vi "Menu Configurator.vi"() -> ()   [LabVIEW 2019, in "Menu Launcher Module.lvlib"]
uses:
  Menu Launcher Module/Menu Launcher Module.lvlib
  <vilib>/National Instruments/Tree Map/Tree Map Data.ctl
  <vilib>/picture/picture.llb/imagedata.ctl
  <vilib>/Utility/miscctls.llb/LVPointTypeDef.ctl
  <vilib>/Utility/miscctls.llb/LVMapReplaceAction.ctl
  <vilib>/National Instruments/Tree Map/API/List Roots.vi
  <vilib>/National Instruments/Tree Map/Utility/Into Tree Control Items.vi
  <vilib>/National Instruments/Tree Map/Tree Map.lvlib
panel:
  in  "New":bool
  in  "Edit":bool
  in  "Save":bool
  in  "Load":bool
  in  "Delete":bool
  in  "Add":bool
  in  "Menu Configuration":string(tree)
  in  "OK":bool
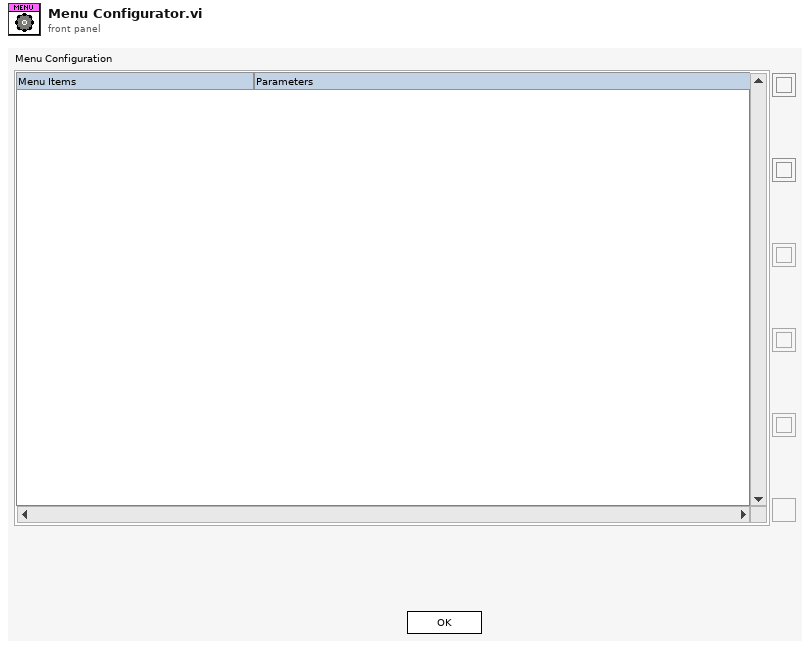
[diagram p1: front panel]
types:
  T1 = enum32{"Invalid", "Standard", "Closed", "Hidden", "Minimized", "Maximized"}
  T2 = enum32{"invalid app kind", "Development System", "Run Time System", "Student Edition", "Embedded LabVIEW", "Evaluation", "Custom"}
  T3 = typedef "Tree Map.lvlib/Tree Map Data.ctl" = map{string, cluster{"Child Paths Set":set{string}, "Name":string, "Data":string, "Attributes":map{string, string}}}
  T4 = typedef "LVPointTypeDef.ctl" = cluster{"Horizontal":i16, "Vertical":i16}
  T5 = enum16{"open", "replace", "create", "open or create", "replace or create", "replace or create with confirmation"}
  T6 = enum8{"Enabled", "Disabled", "Disabled and Grayed Out"}
  T7 = typedef "LVMapReplaceAction.ctl" = enum32{"Modify Entry only if found", "Add or Modify Entry", "Delete Entry"}
  T8 = cluster{"Core":cluster{"Current VI Reference":refnum<vi>, "Close Panel on Exit?":bool}, "SyncSols Menu":T3, "Data Node?":bool, "Path":string, "Selected Tag":string, "Data":string, "Current Path":path}
  T9 = cluster{"Current VI Reference":refnum<vi>, "Close Panel on Exit?":bool}
  T10 = typedef "imagedata.ctl" = cluster{"image type":i32, "image depth":i32, "image":u8[], "mask":u8[], "colors":u32[], "Rectangle":cluster{"left":i16, "top":i16, "right":i16, "bottom":i16}}
  T11 = cluster{"Left Cell String":string, "Child Text":string[], "Child Tag":string, "Item Indent":i32, "Child Only?":bool, "Glyph Index":i32}[]
  T12 = cluster{"Child Paths Set":set{string}, "Name":string, "Data":string, "Attributes":map{string, string}}
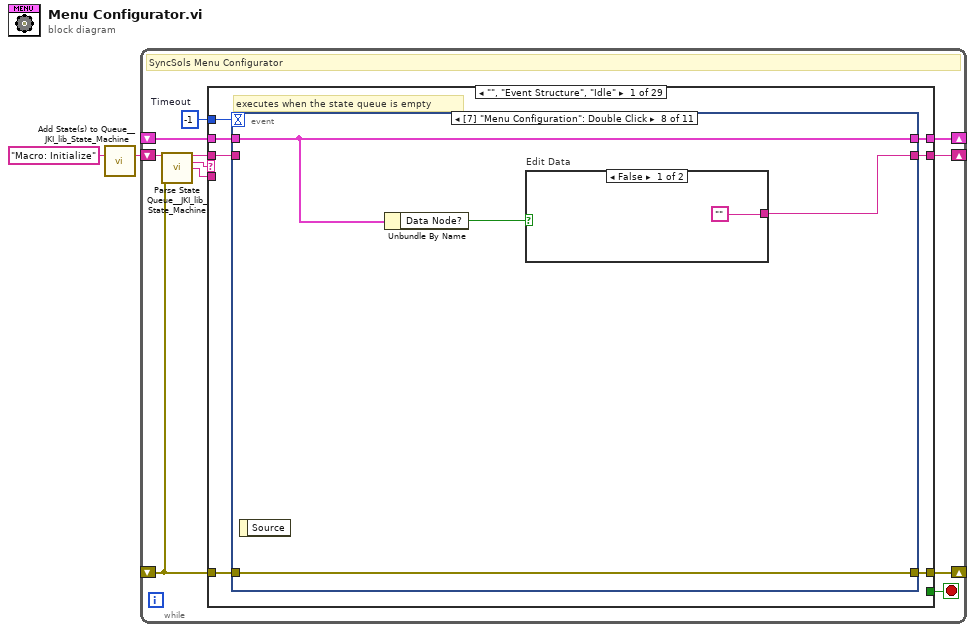
[diagram p0: block diagram]
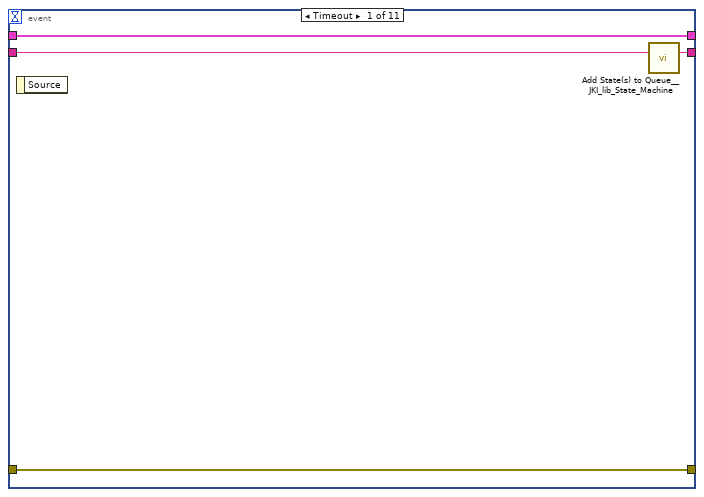
[diagram p2: hidden frame]
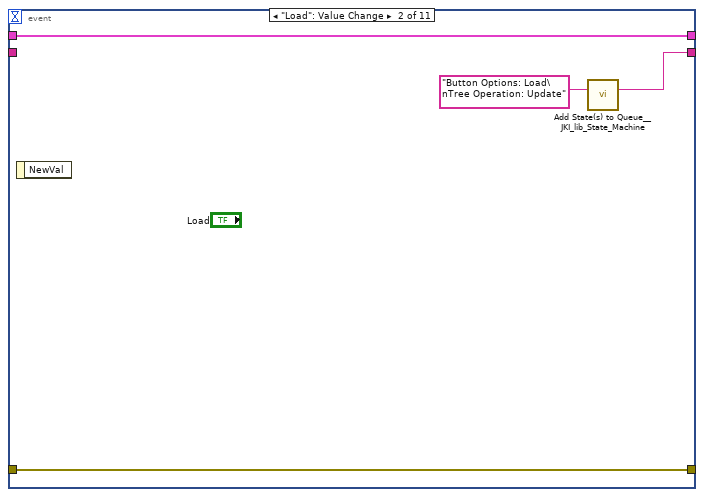
[diagram p3: hidden frame]
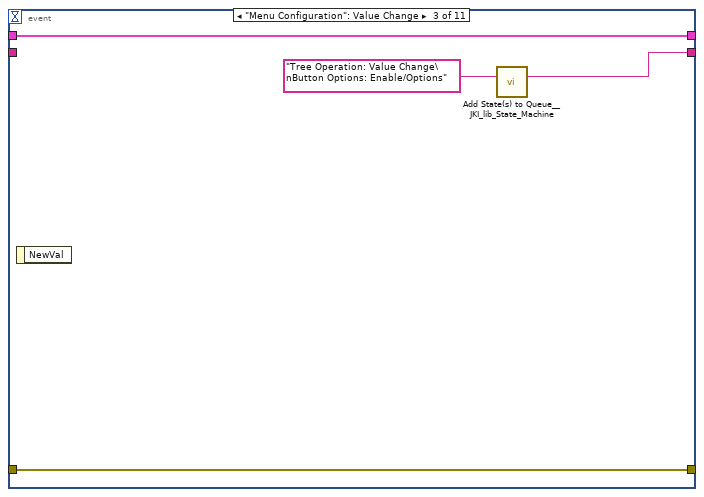
[diagram p4: hidden frame]
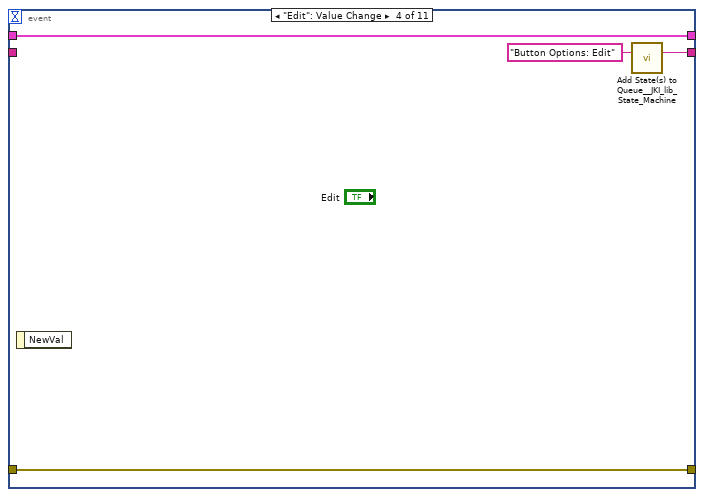
[diagram p5: hidden frame]
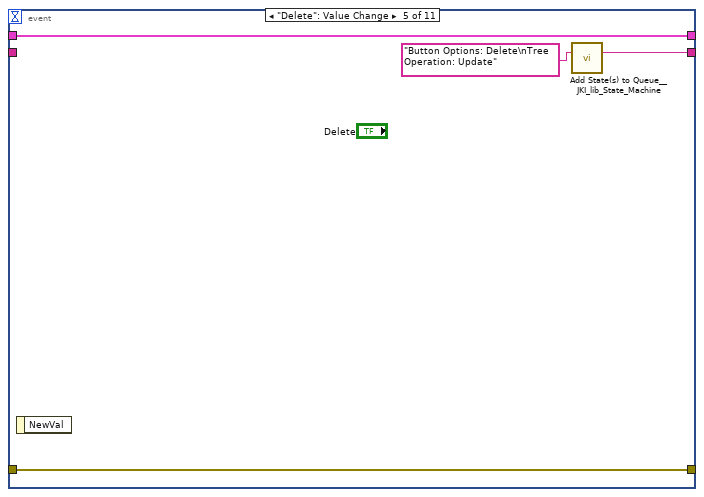
[diagram p6: hidden frame]
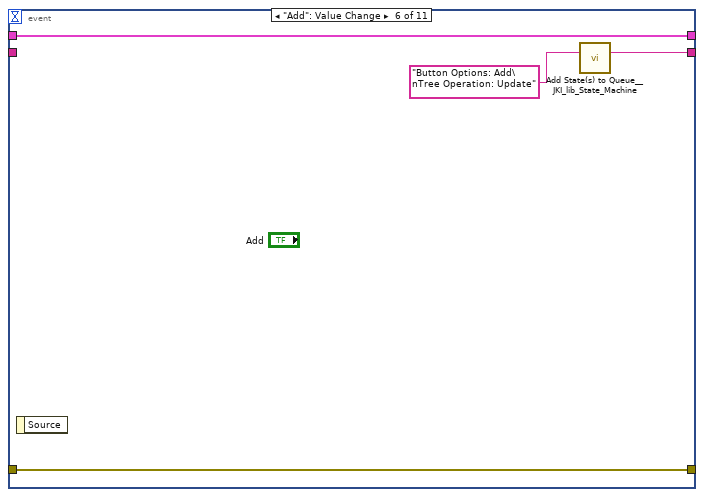
[diagram p7: hidden frame]
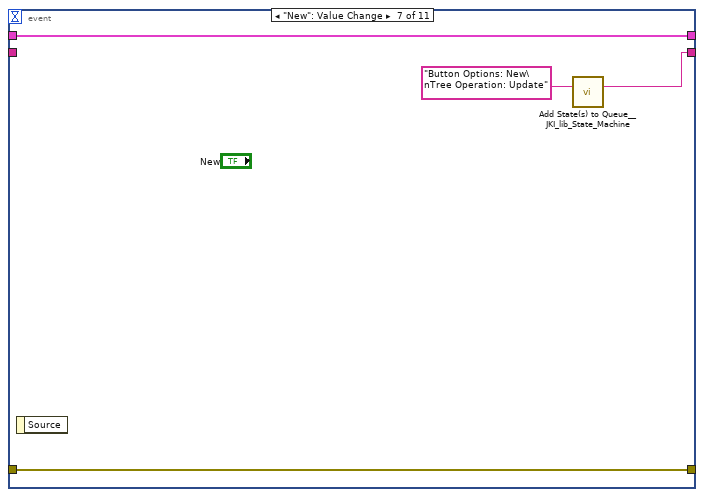
[diagram p8: hidden frame]
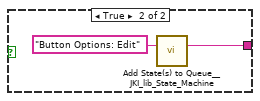
[diagram p9: hidden frame]
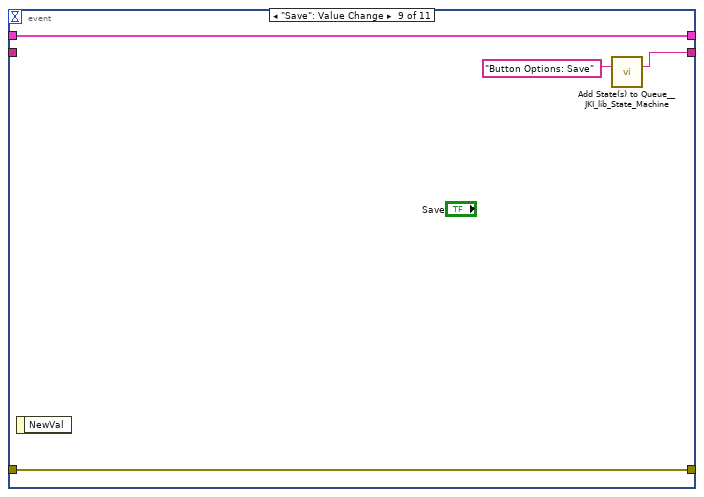
[diagram p10: hidden frame]
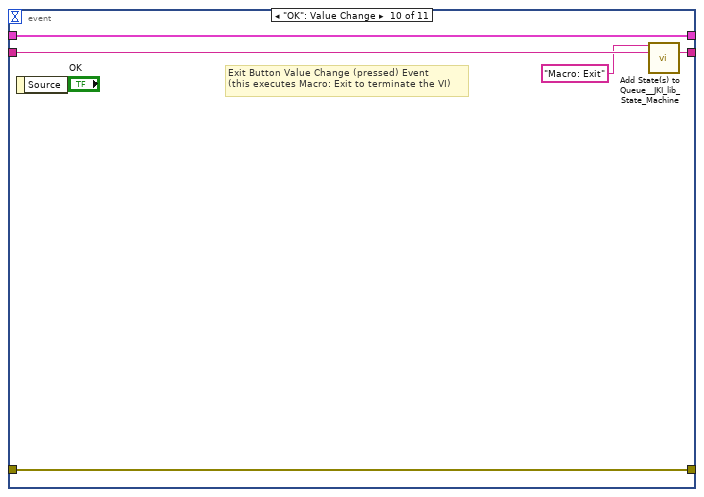
[diagram p11: hidden frame]
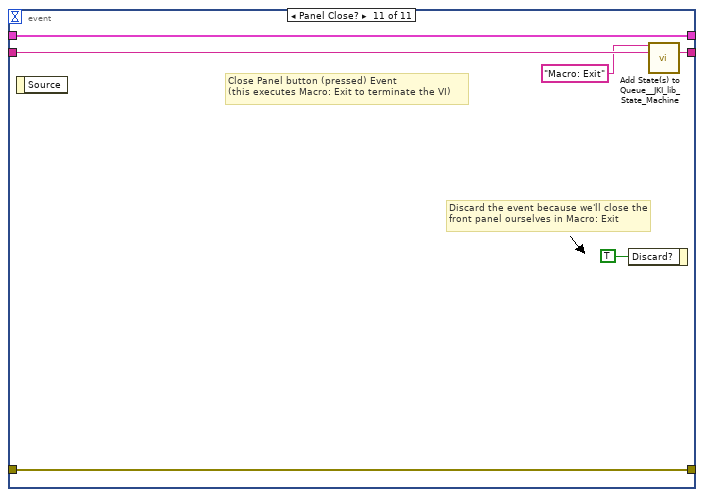
[diagram p12: hidden frame]
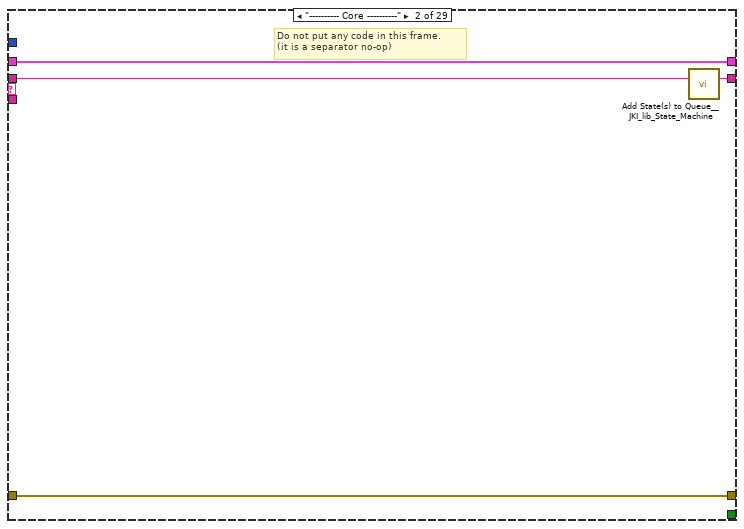
[diagram p13: hidden frame]
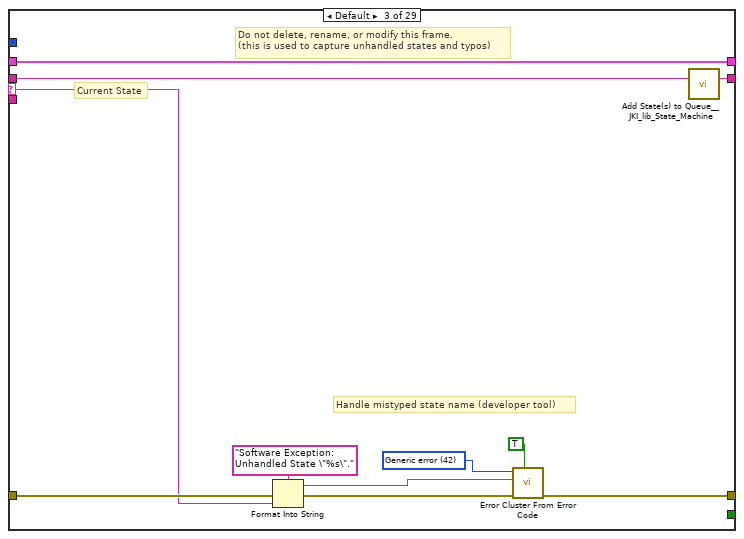
[diagram p14: hidden frame]
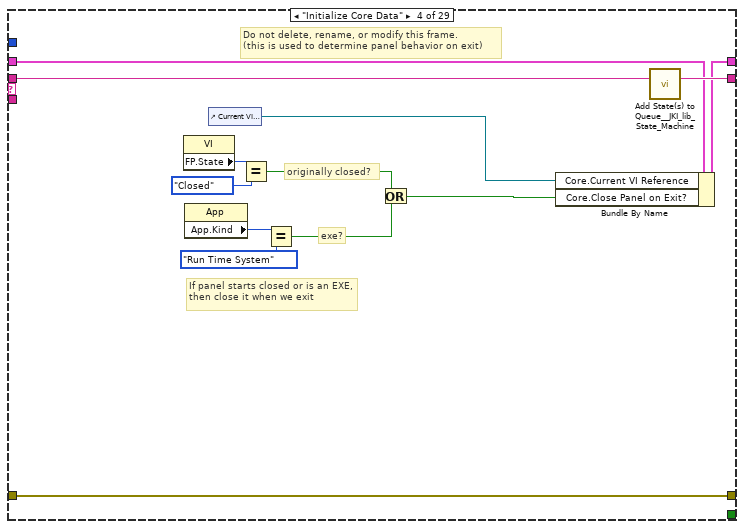
[diagram p15: hidden frame]
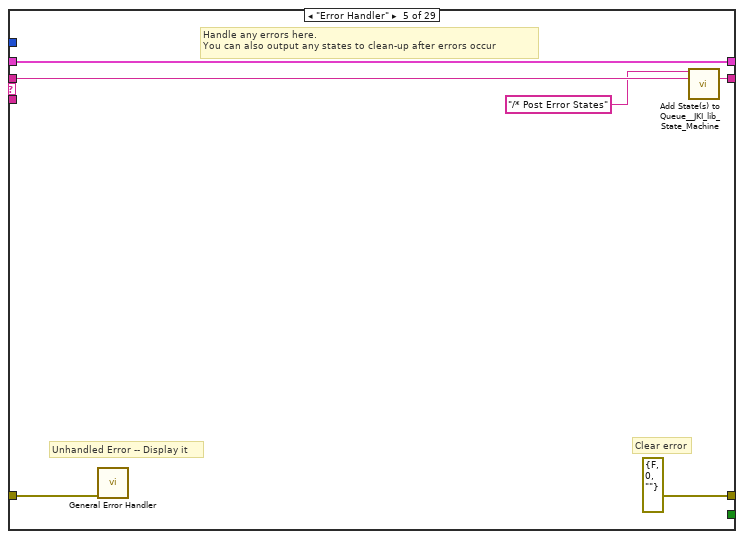
[diagram p16: hidden frame]
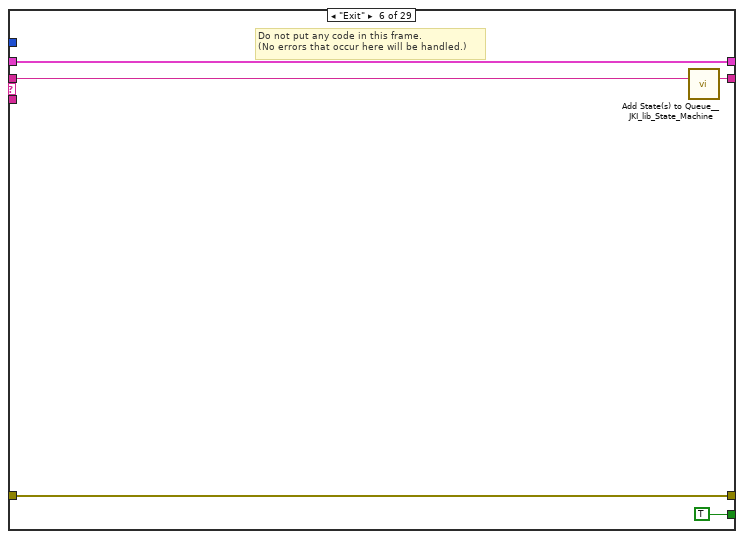
[diagram p17: hidden frame]
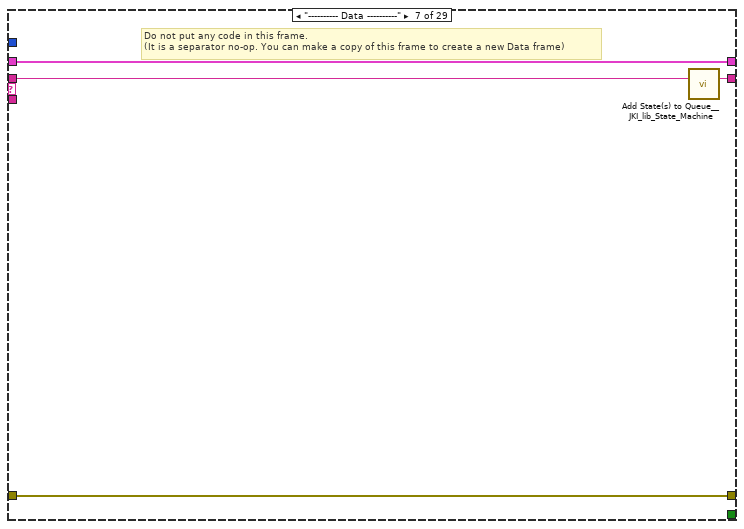
[diagram p18: hidden frame]
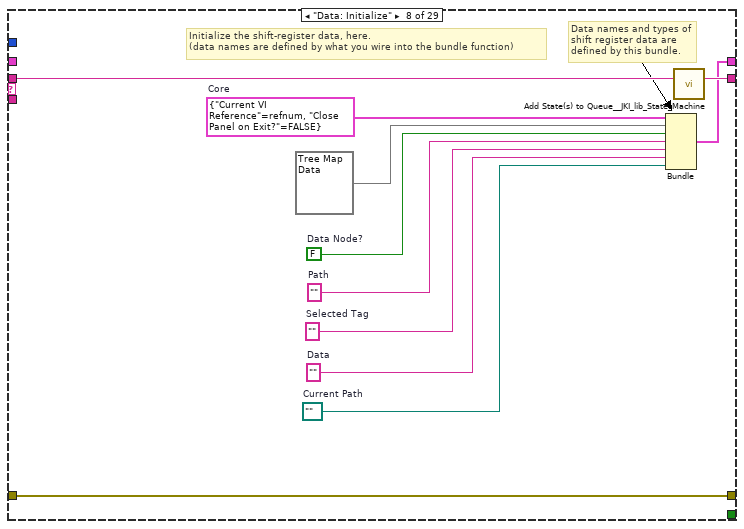
[diagram p19: hidden frame]
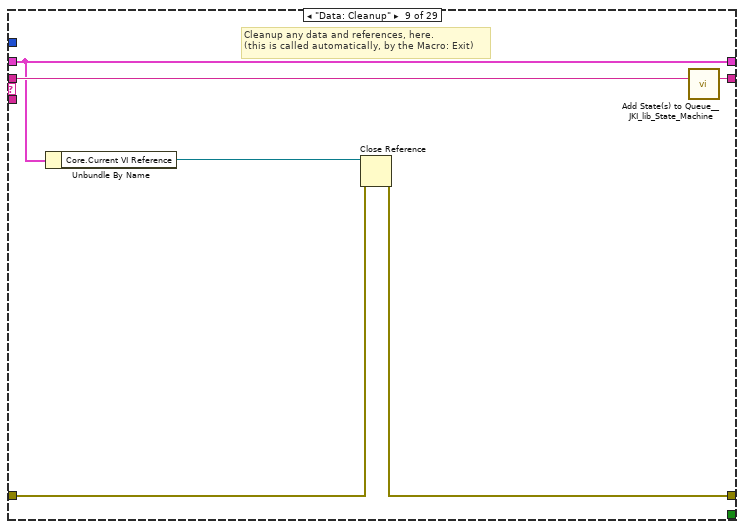
[diagram p20: hidden frame]
diagram:
  n1 = call <vilib>:"Add State(s) to Queue__JKI_lib_State_Machine.vi"("State(s) in (\"\")"="Macro: Initialize") -> ("States Out"=w2:string)  [unwired: 14 in]
  n2 = while "JKI State Machine 2018" {
    shift-right: [w6] -> _
    shift-left: _ -> [w5]
    shift-right: [w9] -> _
    shift-left: _ -> [w3]
    shift-right: [w8] -> _
    shift-left: w2 -> [w10]
    stop <- w7 stop-if-true
    w4 = -1  # Timeout
    # "SyncSols Menu Configurator"
    n3 = call <vilib>:"Parse State Queue__JKI_lib_State_Machine.vi"("State Queue"=w10, "Error In (no error)"=w3) -> ("Remaining States"=w12:string, "Current State"=w13:string, "Arguments"=w11:string)  [unwired: 11 in]
    n4 = case shown="\"\", \"Event Structure\", \"Idle\"" w13 {
      selector: w13 -> [_ _ w75 _ _ _ _ _ _ _ _ _ _ _ _ _ _ _ _ _ _ _ _ _ _ _ _ _ _]
      tunnel: w12 -> [w20 w74 w79 w98 w104 w109 w113 w124 w130 w134 w145 w155 w166 w235 w240 w250 w254 w267 w287 w325 w338 w346 w354 w375 w379 w391 w404 w408 w418]
      tunnel: w11 -> [_ _ _ _ _ _ _ _ _ _ _ w150 w160 _ _ _ _ _ _ _ _ _ _ _ _ _ _ _ _]
      tunnel: w5 -> [w18 w71 w77 w91 w101 w107 w110 _ w125 w131 w143 w153 w162 w232 w237 w247 w251 w257 w285 w323 w336 w343 w352 w372 w376 w389 w401 w405 w415]
      tunnel: [w17 w72 w81 w95 errorcluster {"status"=FALSE, "code"=0, "source"=""} ("error out") w106 w111 w121 w126 w132 w142 w151 w163 w233 w238 w248 w252 w264 w281 w305 w333 w344 w348 w373 w377 w380 w402 w406 w416] -> w9
      tunnel: w3 -> [w16 w72 w80 w95 w100 w106 w111 w121 w127 w132 w142 w152 w164 w233 w238 w248 w252 w265 w281 w318 w334 w344 w348 w373 w377 w385 w402 w406 w416]
      tunnel: [w19 w73 w78 w97 w103 w108 w112 w123 w129 w133 w144 w154 w165 w234 w239 w249 w253 w266 w286 w324 w337 w345 w353 w374 w378 w390 w403 w407 w417] -> w8
      tunnel: [_ _ _ _ _ TRUE _ _ _ _ _ _ _ _ _ _ _ _ _ _ _ _ _ _ _ _ _ _ _] -> w7
      tunnel: [w15 w71 w77 w96 w101 w107 w110 w122 w125 w131 w143 w153 w162 w232 w237 w247 w251 w261 w277 w307 w328 w340 w352 w372 w376 w389 w396 w405 w411] -> w6
      tunnel: w4 -> [w14 _ _ _ _ _ _ _ _ _ _ _ _ _ _ _ _ _ _ _ _ _ _ _ _ _ _ _ _]
      frame "", "Event Structure", "Idle" {
        # "executes when the state queue is empty"
        n5 = event shown="[7] \"Menu Configuration\": Double Click" {
          selector: _ -> [_ _ _ _ _ _ _ _ _ _ _]
          dyn-events: _ -> [_ _ _ _ _ _ _ _ _ _ _]
          timeout: w14 -> [_ _ _ _ _ _ _ _ _ _ _]
          tunnel: w20 -> [w24 _ _ _ _ _ _ _ _ w64 w70]
          tunnel: [w23 w26 w29 w35 w37 w41 w45 w51 w56 w63 w69] -> w19
          tunnel: w18 -> [w21 w28 w30 w36 w40 w44 w48 w52 w59 w61 w67]
          tunnel: [w22 w25 w32 w34 w39 w43 w47 w49 w58 w62 w68] -> w17
          tunnel: w16 -> [w22 w25 w32 w34 w39 w43 w47 w49 w58 w62 w68]
          tunnel: [w21 w28 w30 w36 w40 w44 w48 w52 w59 w61 w67] -> w15
          event Timeout {
            n6 = event-data() -> ()  [unwired: 1 in, 1 out]
            n7 = call <vilib>:"Add State(s) to Queue__JKI_lib_State_Machine.vi"("State(s) in (\"\")"=w24) -> ("States Out"=w23:string)  [unwired: 14 in]
          }
          event "Load": Value Change {
            n8 = event-data() -> ()  [unwired: 1 in, 1 out]
            n9 = call <vilib>:"Add State(s) to Queue__JKI_lib_State_Machine.vi"("State(s) in (\"\")"="Button Options: Load\nTree Operation: Update") -> ("States Out"=w26:string)  [unwired: 14 in]
          }
          event "Menu Configuration": Value Change {
            n10 = event-data() -> ()  [unwired: 1 in, 1 out]
            n11 = call <vilib>:"Add State(s) to Queue__JKI_lib_State_Machine.vi"("State(s) in (\"\")"="Tree Operation: Value Change\nButton Options: Enable/Options") -> ("States Out"=w29:string)  [unwired: 14 in]
          }
          event "Edit": Value Change {
            n12 = event-data() -> ()  [unwired: 1 in, 1 out]
            n13 = call <vilib>:"Add State(s) to Queue__JKI_lib_State_Machine.vi"("State(s) in (\"\")"="Button Options: Edit" ("State(s) in (\"\")")) -> ("States Out"=w35:string)  [unwired: 14 in]
          }
          event "Delete": Value Change {
            n14 = event-data() -> ()  [unwired: 1 in, 1 out]
            n15 = call <vilib>:"Add State(s) to Queue__JKI_lib_State_Machine.vi"("State(s) in (\"\")"="Button Options: Delete\nTree Operation: Update") -> ("States Out"=w37:string)  [unwired: 14 in]
          }
          event "Add": Value Change {
            n16 = event-data() -> ()  [unwired: 1 in, 1 out]
            n17 = call <vilib>:"Add State(s) to Queue__JKI_lib_State_Machine.vi"("State(s) in (\"\")"="Button Options: Add\nTree Operation: Update") -> ("States Out"=w41:string)  [unwired: 14 in]
          }
          event "New": Value Change {
            n18 = event-data() -> ()  [unwired: 1 in, 1 out]
            n19 = call <vilib>:"Add State(s) to Queue__JKI_lib_State_Machine.vi"("State(s) in (\"\")"="Button Options: New\nTree Operation: Update") -> ("States Out"=w45:string)  [unwired: 14 in]
          }
          event "Menu Configuration": Double Click {
            n20 = event-data() -> ()  [unwired: 1 in, 1 out]
            n21 = Unbundle By Name(w52) -> ("Data Node?"=w50:bool)
            n22 = case "Edit Data" shown="False" w50 {
              tunnel: ["" w54] -> w51
              frame False {
              }
              frame True {
                n23 = call <vilib>:"Add State(s) to Queue__JKI_lib_State_Machine.vi"("State(s) in (\"\")"="Button Options: Edit") -> ("States Out"=w54:string)  [unwired: 14 in]
              }
            }
          }
          event "Save": Value Change {
            n24 = event-data() -> ()  [unwired: 1 in, 1 out]
            n25 = call <vilib>:"Add State(s) to Queue__JKI_lib_State_Machine.vi"("State(s) in (\"\")"="Button Options: Save") -> ("States Out"=w56:string)  [unwired: 14 in]
          }
          event "OK": Value Change {
            # "Exit Button Value Change (pressed) Event\n(this executes Macro: Exit to terminate the VI)"
            n26 = event-data() -> ()  [unwired: 1 in, 1 out]
            n27 = call <vilib>:"Add State(s) to Queue__JKI_lib_State_Machine.vi"("State(s) in Front (\"\")"="Macro: Exit", "State(s) in (\"\")"=w64) -> ("States Out"=w63:string)  [unwired: 13 in]
          }
          event Panel Close? {
            # "Discard the event because we'll close the front panel ourselves in Macro: Exit"
            # "Close Panel button (pressed) Event\n(this executes Macro: Exit to terminate the VI)"
            n28 = event-data() -> ()  [unwired: 1 in, 1 out]
            n29 = event-data("Discard?"=TRUE) -> ()  [unwired: 1 in, 1 out]
            n30 = call <vilib>:"Add State(s) to Queue__JKI_lib_State_Machine.vi"("State(s) in Front (\"\")"="Macro: Exit", "State(s) in (\"\")"=w70) -> ("States Out"=w69:string)  [unwired: 13 in]
          }
        }
      }
      frame "---------- Core ----------" {
        # "Do not put any code in this frame.\n(it is a separator no-op)"
        n31 = call <vilib>:"Add State(s) to Queue__JKI_lib_State_Machine.vi"("State(s) in (\"\")"=w74) -> ("States Out"=w73:string)  [unwired: 14 in]
      }
      frame Default {
        w84 = 42 items=["No error", "Argument error", "Memory is full", "Out of zone", "End of file", "File already open", "Generic file I/O error", "File not found", "File permission error", "Disk is full", "Duplicate path", "Too many files open", "System feature not enabled", "Resource file not found", "Cannot add resource", "Resource not found", "Image not found", "Image memory error", "Pen does not exist", "Config type invalid", "Config token not found", "Config parse error", "Config memory error", "Bad external code format", "Bad external code offset", "External code not present", "Null window", "Destroy window error", "Null menu", "Print aborted", "Bad print record", "Print driver error", "Windows error during printing", "Memory error during printing", "Print dialog error", "Generic print error", "Invalid device refnum", "Device not found", "Device parameter error", "Device unit error", "Cannot open device", "Device call aborted", "Generic error", "Cancelled by user", "Object ID too low", "Object ID too high", "Object not in heap", "Unknown heap", "Unknown object (invalid DefProc)", "Unknown object (DefProc not in table)", "Message out of range", "Invalid (null) method", "Unknown message", "Manager call not supported", "Bad address", "Network operation in progress", "Network operation timed out", "Connection is busy", "Network attribute not supported", "Network error", "Address in use", "System out of memory", "Connection aborted", "Connection refused", "Not connected", "Already connected", "Connection closed", "Initialization error (interapplication manager)", "Bad occurrence", "Wait on unbound occurrence handler", "Occurrence queue overflow", "Datalog type conflict", "Unused", "Unrecognized type (interapplication manager)", "Memory corrupt", "Failed to make temporary DLL", "Old CIN version", "Drag socket not found", "Failed to load drop-object", "Failed to register OLE object", "Failed to release OLE object", "Format specifier type mismatch", "Unknown format specifier", "Too few format specifiers", "Too many format specifiers", "Scan failed", "Newer CIN version", "Error converting to variant", "Runtime menu error", "Password tampered", "Variant attribute not found", "Incompatible variant data type", "Event data is not available", "Event Store is not present", "Occurrence is not found", "Event Queue is not created", "Event info is not available", "Refnum passed is NULL", "Error retrieving Class GUID", "Error retrieving CoClass GUID", "Error retrieving TypeLib GUID.", "Bad built application magic bytes.", "Specific driver is different from the specific driver associated with the Logical Name.", "There is no session opened to the class driver.", "Max Error", "MAX - Error with config objects", "MAX - Error loading configuration", "MAX - Group not supported"]
        # "Current State"
        # "Do not delete, rename, or modify this frame.\n(this is used to capture unhandled states and typos)"
        # "Handle mistyped state name (developer tool)"
        n32 = Format Into String(format string="Software Exception: Unhandled State \"%s\"." ("message"), error in=w80, w75) -> (resulting string=w83:string, error out=w82:errorcluster)  [unwired: 1 in]
        n33 = call <vilib>:"Error Cluster From Error Code.vi"("show call chain? (False)"=TRUE, "error in (no error)"=w82, "error message (\"\")"=w83, "error code (0)"=w84) -> ("error out"=w81:errorcluster)  [unwired: 5 in]
        n34 = call <vilib>:"Add State(s) to Queue__JKI_lib_State_Machine.vi"("State(s) in (\"\")"=w79) -> ("States Out"=w78:string)  [unwired: 14 in]
      }
      frame "Initialize Core Data" {
        # "Do not delete, rename, or modify this frame.\n(this is used to determine panel behavior on exit)"
        # "originally closed?"
        # "exe?"
        # "If panel starts closed or is an EXE, then close it when we exit"
        n35 = property class="VI"() -> ("FP.State"=w88:T1)  [unwired: 2 in, 2 out]
        n36 = property class="App"() -> ("App.Kind"=w94:T2)  [unwired: 2 in, 2 out]
        n37 = control-ref of="Current VI Reference"() -> (w89:refnum<vi>)
        n38 = Equal?(x=w88, y=T1."Closed" ("Front Panel Window:State")) -> (x = y?=w86:bool)
        n39 = Equal?(x=w94, y=T2."Run Time System" ("Application:Kind")) -> (x = y?=w92:bool)
        n40 = Or(x=w86, y=w92) -> (x .or. y?=w90:bool)
        n41 = Bundle By Name(cluster=w91, "Core.Current VI Reference"=w89, "Core.Close Panel on Exit?"=w90) -> (w96:T8)
        n42 = call <vilib>:"Add State(s) to Queue__JKI_lib_State_Machine.vi"("State(s) in (\"\")"=w98) -> ("States Out"=w97:string)  [unwired: 14 in]
      }
      frame "Error Handler" {
        # "Unhandled Error -- Display it"
        # "Handle any errors here.\nYou can also output any states to clean-up after errors occur"
        # "Clear error"
        n43 = call <vilib>:"General Error Handler.vi"("error in (no error)"=w100) -> ()  [unwired: 10 in, 5 out]
        n44 = call <vilib>:"Add State(s) to Queue__JKI_lib_State_Machine.vi"("State(s) in Front (\"\")"="/* Post Error States", "State(s) in (\"\")"=w104) -> ("States Out"=w103:string)  [unwired: 13 in]
      }
      frame "Exit" {
        # "Do not put any code in this frame.\n(No errors that occur here will be handled.)"
        n45 = call <vilib>:"Add State(s) to Queue__JKI_lib_State_Machine.vi"("State(s) in (\"\")"=w109) -> ("States Out"=w108:string)  [unwired: 14 in]
      }
      frame "---------- Data ----------" {
        # "Do not put any code in this frame.\n(It is a separator no-op. You can make a copy of this frame to create a new Data frame)"
        n46 = call <vilib>:"Add State(s) to Queue__JKI_lib_State_Machine.vi"("State(s) in (\"\")"=w113) -> ("States Out"=w112:string)  [unwired: 14 in]
      }
      frame "Data: Initialize" {
        w114 = path ""  # Current Path
        w115 = ""  # Data
        w116 = ""  # Selected Tag
        w117 = ""  # Path
        w118 = FALSE  # Data Node?
        w120 = T9 {"Current VI Reference"=refnum, "Close Panel on Exit?"=FALSE}  # Core
        # "Data names and types of shift register data are defined by this bundle."
        # "Initialize the shift-register data, here.\n(data names are defined by what you wire into the bundle function)"
        n47 = Bundle("Core"=w120, "SyncSols Menu"=T3 {}, "Data Node?"=w118, "Path"=w117, "Selected Tag"=w116, "Data"=w115, "Current Path"=w114) -> (w122:T8)  [unwired: 1 in]
        n48 = call <vilib>:"Add State(s) to Queue__JKI_lib_State_Machine.vi"("State(s) in (\"\")"=w124) -> ("States Out"=w123:string)  [unwired: 14 in]
      }
      frame "Data: Cleanup" {
        # "Cleanup any data and references, here.\n(this is called automatically, by the Macro: Exit)"
        n49 = Unbundle By Name(w125) -> ("Core.Current VI Reference"=w128:refnum<vi>)
        n50 = Close Reference(reference=w128, error in (no error)=w127) -> (error out=w126:errorcluster)
        n51 = call <vilib>:"Add State(s) to Queue__JKI_lib_State_Machine.vi"("State(s) in (\"\")"=w130) -> ("States Out"=w129:string)  [unwired: 14 in]
      }
      frame "---------- UI ----------" {
        # "Do not put any code in this frame.\n(It is a separator no-op. You can make a copy of this frame to create a new UI frame)"
        n52 = call <vilib>:"Add State(s) to Queue__JKI_lib_State_Machine.vi"("State(s) in (\"\")"=w134) -> ("States Out"=w133:string)  [unwired: 14 in]
      }
      frame "UI: Initialize" {
        w136 = T10 {"image type"=0, "image depth"=32, "image"=[0, 0, 0, 0, 0, 0, 0, 0, 0, 0, 0, 0, 0, 0, 0, 0, 1, 0, 0, 0, 1, 0, 0, 0, 3, 60, 60, 60, 3, 84, 84, 84, 3, 95, 95, 95, 3, 75, 75, 75, 2, 157, 157, 157, 1, 166, 166, 166, 0, 0, 0, 0, 0, 0, 0, 0, 0, 0, 0, 0, 0, 0, 0, 0, 0, 0, 0, 0, 0, 0, 0, 0, 0, 0, 0, 0, 1, 1, 1, 1, 3, 131, 131, 131, 6, 236, 236, 236, 9, 255, 255, 255, 11, 255, 255, 255, 11, 255, 255, 255, 10, 255, 255, 255, 50, 254, 254, 254, 64, 251, 251, 251, 2, 165, 164, 165, 0, 0, 0, 0, 0, 0, 0, 0, 0, 0, 0, 0, 0, 0, 0, 0, 0, 0, 0, 0, 1, 2, 2, 2, 4, 170, 171, 171, 9, 252, 254, 254, 27, 242, 245, 251, 91, 249, 211, 230, 122, 253, 196, 219, 114, 254, 199, 221, 66, 252, 229, 239, 182, 234, 234, 234, 252, 221, 220, 219, 134, 185, 185, 184, 7, 241, 240, 241, 0, 0, 0, 0, 0, 0, 0, 0, 0, 0, 0, 0, 1, 0, 0, 0, 3, 114, 116, 117, 11, 235, 246, 253, 127, 225, 180, 215, 241, 251, 122, 176, 255, 255, 111, 168, 255, 255, 117, 173, 255, 255, 119, 174, 254, 254, 141, 187, 249, 245, 149, 189, 251, 190, 167, 175, 219, 184, 182, 182, 11, 221, 220, 221, 2, 47, 47, 47, 0, 0, 0, 0, 0, 0, 0, 0, 1, 7, 8, 9, 6, 174, 204, 226, 164, 218, 141, 192, 255, 255, 108, 166, 255, 255, 116, 171, 255, 255, 128, 180, 255, 255, 139, 187, 255, 255, 135, 184, 255, 255, 154, 196, 255, 255, 161, 201, 254, 251, 134, 181, 152, 250, 232, 239, 15, 254, 254, 254, 3, 135, 135, 135, 0, 0, 0, 0, 0, 0, 0, 0, 2, 41, 62, 77, 98, 181, 154, 208, 255, 255, 90, 153, 255, 255, 100, 160, 255, 255, 117, 172, 255, 255, 142, 189, 255, 255, 158, 199, 255, 255, 157, 198, 255, 255, 176, 209, 255, 255, 174, 208, 255, 255, 142, 188, 226, 253, 104, 160, 32, 253, 247, 250, 7, 247, 247, 247, 1, 35, 35, 35, 0, 0, 0, 0, 2, 74, 69, 105, 214, 233, 79, 146, 255, 255, 78, 143, 255, 255, 89, 152, 255, 255, 119, 174, 255, 255, 144, 190, 255, 255, 160, 200, 255, 255, 186, 215, 255, 255, 186, 215, 255, 255, 172, 207, 255, 255, 155, 197, 255, 255, 95, 156, 109, 251, 174, 201, 8, 255, 255, 255, 2, 37, 37, 37, 0, 0, 0, 0, 26, 118, 63, 111, 254, 254, 56, 124, 255, 255, 61, 128, 255, 255, 81, 146, 255, 255, 115, 170, 255, 255, 133, 183, 255, 255, 153, 196, 255, 255, 180, 212, 255, 255, 181, 212, 255, 255, 168, 204, 255, 255, 134, 184, 255, 255, 96, 157, 173, 252, 120, 166, 9, 255, 255, 255, 2, 44, 44, 44, 0, 0, 0, 0, 48, 128, 67, 116, 255, 252, 50, 117, 255, 253, 60, 126, 255, 255, 70, 136, 255, 255, 90, 152, 255, 255, 113, 169, 255, 255, 127, 179, 255, 255, 144, 190, 255, 255, 160, 200, 255, 255, 135, 184, 255, 255, 102, 162, 255, 255, 73, 139, 194, 253, 102, 154, 9, 255, 255, 255, 2, 47, 47, 47, 0, 0, 0, 0, 27, 119, 59, 106, 254, 249, 48, 115, 255, 242, 42, 106, 255, 254, 57, 125, 255, 255, 71, 138, 255, 255, 81, 145, 255, 255, 92, 155, 255, 255, 102, 162, 255, 255, 103, 162, 255, 255, 95, 156, 255, 255, 76, 142, 255, 255, 65, 132, 176, 251, 114, 162, 7, 254, 254, 255, 1, 26, 26, 26, 0, 0, 0, 0, 0, 0, 0, 0, 216, 240, 60, 128, 255, 232, 38, 99, 255, 247, 47, 112, 255, 253, 57, 124, 255, 255, 65, 132, 255, 255, 64, 132, 255, 255, 75, 140, 255, 255, 73, 138, 255, 255, 66, 133, 255, 255, 68, 134, 255, 255, 59, 126, 114, 243, 165, 199, 4, 190, 191, 193, 1, 0, 0, 0, 0, 0, 0, 0, 0, 0, 0, 0, 99, 213, 67, 137, 255, 237, 41, 104, 255, 221, 34, 91, 255, 233, 38, 100, 255, 243, 44, 108, 255, 250, 46, 112, 255, 252, 50, 117, 255, 254, 48, 116, 255, 255, 53, 120, 255, 255, 69, 135, 235, 246, 72, 137, 21, 206, 218, 240, 2, 48, 50, 51, 0, 0, 0, 0, 0, 0, 0, 0, 0, 0, 0, 0, 1, 86, 29, 70, 169, 222, 46, 115, 255, 219, 33, 90, 255, 210, 31, 85, 255, 218, 33, 90, 255, 228, 36, 96, 255, 237, 39, 101, 255, 247, 43, 109, 255, 254, 53, 121, 249, 250, 63, 130, 78, 166, 162, 217, 2, 91, 117, 134, 1, 0, 0, 0, 0, 0, 0, 0, 0, 0, 0, 0, 0, 0, 0, 0, 0, 0, 0, 0, 4, 93, 29, 77, 133, 213, 48, 118, 247, 225, 38, 98, 255, 207, 29, 82, 255, 213, 32, 86, 255, 223, 34, 92, 255, 237, 42, 104, 220, 222, 71, 142, 68, 121, 137, 218, 1, 60, 110, 153, 0, 0, 0, 0, 0, 0, 0, 0, 0, 0, 0, 0, 0, 0, 0, 0, 0, 0, 0, 0, 0, 0, 0, 0, 0, 0, 0, 0, 0, 0, 0, 0, 22, 125, 46, 103, 96, 187, 60, 131, 131, 207, 64, 135, 123, 202, 73, 148, 71, 132, 92, 180, 5, 49, 86, 165, 0, 0, 0, 0, 0, 0, 0, 0, 0, 0, 0, 0, 0, 0, 0, 0, 0, 0, 0, 0, 0, 0, 0, 0, 0, 0, 0, 0, 0, 0, 0, 0, 0, 0, 0, 0, 0, 0, 0, 0, 0, 0, 0, 0, 0, 0, 0, 0, 0, 0, 0, 0, 0, 0, 0, 0, 0, 0, 0, 0, 0, 0, 0, 0, 0, 0, 0, 0, 0, 0, 0, 0, 0, 0, 0, 0, 0, 0, 0, 0, 0, 0, 0, 0], "mask"=[0, 0, 0, 0, 0, 56, 15, 248, 31, 248, 31, 248, 63, 248, 63, 252, 63, 252, 63, 252, 63, 248, 31, 248, 31, 240, 15, 224, 1, 0, 0, 0], "colors"=[], "Rectangle"={"left"=0, "top"=0, "right"=16, "bottom"=16}}  # Red Ball
        w137 = T10 {"image type"=0, "image depth"=32, "image"=[0, 0, 0, 0, 0, 0, 0, 0, 0, 0, 0, 0, 0, 0, 0, 0, 1, 0, 0, 0, 1, 0, 0, 0, 3, 60, 60, 60, 3, 84, 84, 84, 3, 95, 95, 95, 3, 75, 75, 75, 2, 157, 157, 157, 1, 166, 166, 166, 0, 0, 0, 0, 0, 0, 0, 0, 0, 0, 0, 0, 0, 0, 0, 0, 0, 0, 0, 0, 0, 0, 0, 0, 0, 0, 0, 0, 1, 1, 1, 1, 3, 131, 131, 131, 6, 236, 236, 236, 9, 255, 255, 255, 11, 255, 255, 255, 11, 255, 255, 255, 10, 255, 255, 255, 50, 254, 254, 254, 64, 251, 251, 251, 2, 165, 164, 165, 0, 0, 0, 0, 0, 0, 0, 0, 0, 0, 0, 0, 0, 0, 0, 0, 0, 0, 0, 0, 1, 2, 2, 2, 4, 170, 171, 171, 9, 252, 254, 254, 27, 237, 248, 253, 90, 201, 234, 252, 122, 183, 227, 252, 113, 188, 229, 251, 65, 224, 242, 251, 182, 234, 234, 234, 252, 221, 220, 219, 134, 185, 185, 184, 7, 241, 240, 241, 0, 0, 0, 0, 0, 0, 0, 0, 0, 0, 0, 0, 1, 0, 0, 0, 3, 114, 116, 117, 11, 234, 246, 254, 126, 148, 215, 251, 241, 87, 192, 252, 255, 74, 188, 255, 255, 80, 191, 255, 255, 83, 192, 255, 254, 109, 202, 254, 249, 125, 202, 244, 250, 162, 179, 188, 219, 184, 182, 182, 11, 221, 220, 221, 2, 47, 47, 47, 0, 0, 0, 0, 0, 0, 0, 0, 1, 7, 8, 9, 6, 171, 206, 227, 163, 98, 194, 249, 255, 71, 187, 254, 255, 79, 191, 255, 255, 91, 197, 255, 255, 104, 202, 255, 255, 99, 201, 255, 255, 122, 209, 255, 255, 129, 214, 255, 254, 104, 198, 251, 151, 229, 242, 250, 15, 254, 254, 254, 3, 135, 135, 135, 0, 0, 0, 0, 0, 0, 0, 0, 2, 38, 64, 78, 97, 97, 191, 248, 255, 52, 179, 253, 255, 61, 184, 254, 255, 78, 192, 255, 255, 106, 205, 255, 255, 125, 213, 255, 255, 123, 213, 255, 255, 147, 221, 255, 255, 144, 220, 255, 255, 106, 206, 255, 226, 72, 184, 253, 32, 246, 250, 253, 7, 247, 247, 247, 1, 35, 35, 35, 0, 0, 0, 0, 2, 34, 88, 124, 213, 39, 163, 249, 255, 41, 170, 252, 255, 50, 178, 254, 255, 80, 195, 255, 255, 107, 207, 255, 255, 126, 214, 255, 255, 157, 226, 255, 255, 159, 226, 255, 255, 140, 220, 255, 255, 118, 213, 255, 255, 54, 183, 255, 108, 161, 213, 251, 8, 255, 255, 255, 2, 37, 37, 37, 0, 0, 0, 0, 26, 33, 103, 151, 254, 25, 154, 249, 255, 27, 158, 251, 255, 43, 174, 254, 255, 75, 193, 255, 255, 94, 202, 255, 255, 117, 212, 255, 255, 150, 223, 255, 255, 151, 224, 255, 255, 133, 219, 255, 255, 95, 204, 255, 255, 54, 185, 255, 172, 98, 188, 252, 9, 255, 255, 255, 2, 44, 44, 44, 0, 0, 0, 0, 47, 36, 110, 161, 255, 20, 147, 245, 255, 28, 156, 248, 255, 34, 167, 253, 255, 50, 180, 254, 255, 73, 193, 255, 255, 87, 200, 255, 255, 107, 208, 255, 255, 124, 216, 255, 255, 93, 205, 255, 255, 60, 189, 255, 255, 34, 171, 255, 194, 78, 178, 253, 9, 255, 255, 255, 2, 47, 47, 47, 0, 0, 0, 0, 26, 32, 101, 148, 254, 20, 145, 243, 255, 15, 138, 242, 255, 24, 157, 251, 255, 33, 169, 254, 255, 41, 175, 255, 255, 51, 182, 255, 255, 61, 188, 255, 255, 61, 189, 255, 255, 53, 185, 255, 255, 36, 174, 255, 255, 28, 165, 255, 175, 92, 183, 253, 7, 254, 254, 255, 1, 26, 26, 26, 0, 0, 0, 0, 0, 0, 0, 0, 215, 29, 151, 243, 255, 12, 130, 235, 255, 17, 145, 246, 255, 23, 157, 252, 255, 29, 164, 254, 255, 27, 165, 255, 255, 35, 172, 255, 255, 34, 170, 255, 255, 28, 166, 255, 255, 30, 167, 255, 255, 24, 159, 255, 113, 145, 209, 254, 4, 190, 191, 193, 1, 0, 0, 0, 0, 0, 0, 0, 0, 0, 0, 0, 98, 32, 148, 234, 255, 15, 133, 236, 255, 9, 123, 235, 255, 11, 135, 245, 255, 14, 144, 251, 255, 15, 148, 253, 255, 18, 152, 254, 255, 16, 152, 255, 255, 19, 155, 255, 255, 32, 167, 255, 234, 37, 163, 254, 21, 187, 227, 250, 2, 48, 50, 51, 0, 0, 0, 0, 0, 0, 0, 0, 0, 0, 0, 0, 1, 10, 63, 112, 168, 15, 137, 241, 255, 9, 122, 234, 255, 8, 117, 234, 255, 8, 125, 242, 255, 9, 133, 248, 255, 10, 138, 252, 255, 14, 145, 253, 255, 21, 155, 254, 249, 27, 160, 254, 77, 97, 194, 254, 2, 87, 119, 136, 1, 0, 0, 0, 0, 0, 0, 0, 0, 0, 0, 0, 0, 0, 0, 0, 0, 0, 0, 0, 3, 8, 69, 128, 132, 16, 133, 239, 247, 12, 128, 240, 255, 6, 116, 236, 255, 7, 121, 240, 255, 8, 128, 246, 255, 13, 139, 251, 219, 29, 155, 253, 67, 55, 167, 254, 1, 54, 114, 157, 0, 0, 0, 0, 0, 0, 0, 0, 0, 0, 0, 0, 0, 0, 0, 0, 0, 0, 0, 0, 0, 0, 0, 0, 0, 0, 0, 0, 0, 0, 0, 0, 21, 19, 98, 167, 95, 26, 134, 229, 130, 29, 145, 244, 122, 33, 149, 247, 70, 31, 139, 236, 5, 21, 100, 181, 0, 0, 0, 0, 0, 0, 0, 0, 0, 0, 0, 0, 0, 0, 0, 0, 0, 0, 0, 0, 0, 0, 0, 0, 0, 0, 0, 0, 0, 0, 0, 0, 0, 0, 0, 0, 0, 0, 0, 0, 0, 0, 0, 0, 0, 0, 0, 0, 0, 0, 0, 0, 0, 0, 0, 0, 0, 0, 0, 0, 0, 0, 0, 0, 0, 0, 0, 0, 0, 0, 0, 0, 0, 0, 0, 0, 0, 0, 0, 0, 0, 0, 0, 0], "mask"=[0, 0, 0, 0, 0, 56, 7, 248, 31, 248, 31, 248, 63, 248, 63, 252, 63, 252, 63, 252, 63, 248, 31, 248, 31, 240, 15, 224, 1, 0, 0, 0], "colors"=[], "Rectangle"={"left"=0, "top"=0, "right"=16, "bottom"=16}}  # Blue Ball
        w139 = T10 {"image type"=0, "image depth"=32, "image"=[0, 0, 0, 0, 0, 0, 0, 0, 0, 0, 0, 0, 0, 0, 0, 0, 0, 0, 0, 0, 0, 0, 0, 0, 0, 0, 0, 0, 0, 0, 0, 0, 0, 0, 0, 0, 0, 0, 0, 0, 0, 1, 0, 0, 0, 1, 1, 0, 0, 1, 1, 0, 0, 1, 1, 0, 0, 1, 1, 0, 0, 1, 0, 0, 0, 0, 0, 0, 0, 0, 0, 0, 0, 1, 0, 0, 0, 1, 0, 0, 0, 1, 0, 0, 0, 1, 0, 0, 0, 1, 0, 0, 0, 1, 0, 0, 0, 2, 1, 0, 1, 17, 14, 2, 9, 79, 67, 14, 20, 88, 74, 15, 21, 88, 74, 15, 21, 88, 74, 15, 19, 88, 73, 15, 1, 47, 39, 8, 1, 26, 18, 4, 2, 63, 43, 10, 2, 64, 43, 10, 2, 64, 43, 10, 2, 64, 43, 10, 2, 64, 43, 10, 2, 64, 43, 10, 2, 64, 43, 10, 5, 86, 64, 14, 145, 227, 191, 40, 245, 249, 208, 43, 252, 249, 209, 43, 252, 249, 209, 43, 252, 249, 209, 43, 252, 249, 209, 43, 174, 244, 204, 42, 140, 223, 150, 36, 249, 242, 163, 40, 252, 242, 163, 40, 252, 242, 163, 40, 252, 242, 163, 40, 252, 242, 163, 40, 252, 242, 163, 40, 252, 242, 164, 40, 253, 246, 187, 41, 253, 250, 209, 42, 254, 251, 210, 42, 254, 252, 211, 42, 255, 252, 211, 42, 255, 252, 211, 42, 254, 251, 210, 42, 253, 251, 210, 42, 232, 238, 158, 33, 254, 238, 158, 33, 254, 239, 159, 34, 255, 239, 159, 34, 255, 239, 159, 34, 255, 239, 159, 34, 255, 239, 159, 34, 255, 242, 169, 36, 255, 250, 208, 40, 255, 250, 209, 40, 255, 251, 209, 41, 255, 251, 209, 41, 255, 251, 209, 41, 255, 251, 209, 41, 254, 251, 209, 41, 254, 251, 209, 41, 235, 232, 152, 27, 254, 233, 155, 28, 255, 233, 156, 28, 255, 233, 156, 28, 255, 233, 156, 28, 255, 233, 157, 28, 255, 238, 171, 32, 255, 247, 202, 37, 255, 249, 207, 38, 255, 250, 208, 39, 255, 250, 208, 39, 255, 250, 208, 39, 255, 250, 208, 39, 255, 250, 208, 39, 255, 250, 208, 39, 255, 250, 208, 39, 236, 241, 187, 32, 254, 248, 205, 36, 255, 248, 206, 36, 255, 248, 206, 36, 255, 248, 206, 36, 255, 248, 206, 36, 255, 248, 206, 36, 255, 248, 206, 36, 255, 248, 206, 36, 255, 249, 207, 37, 255, 249, 207, 37, 255, 249, 207, 37, 255, 249, 207, 37, 255, 249, 207, 37, 255, 249, 207, 37, 255, 249, 207, 37, 253, 247, 205, 34, 254, 247, 205, 34, 255, 248, 206, 35, 255, 248, 206, 35, 255, 248, 206, 35, 255, 248, 206, 35, 255, 248, 206, 35, 255, 248, 206, 35, 255, 248, 206, 35, 255, 248, 206, 35, 255, 248, 206, 35, 255, 248, 206, 35, 255, 248, 206, 35, 255, 248, 206, 35, 255, 248, 206, 35, 255, 248, 206, 35, 254, 247, 205, 33, 254, 247, 205, 33, 255, 247, 205, 33, 255, 247, 205, 33, 255, 247, 205, 33, 255, 247, 205, 33, 255, 247, 205, 33, 255, 247, 205, 33, 255, 247, 205, 33, 255, 247, 205, 33, 255, 247, 205, 33, 255, 247, 205, 33, 255, 247, 205, 33, 255, 247, 205, 33, 255, 247, 205, 33, 255, 247, 205, 33, 255, 246, 204, 32, 255, 246, 204, 32, 255, 246, 204, 32, 255, 246, 204, 32, 255, 246, 204, 32, 255, 246, 204, 32, 255, 246, 204, 32, 255, 246, 204, 32, 255, 246, 204, 32, 255, 246, 204, 32, 255, 246, 204, 32, 255, 246, 204, 32, 255, 246, 204, 32, 255, 246, 204, 32, 255, 246, 204, 32, 255, 246, 204, 32, 255, 245, 203, 30, 255, 245, 203, 30, 255, 245, 203, 30, 255, 245, 203, 30, 255, 245, 203, 30, 255, 245, 203, 30, 255, 245, 203, 30, 255, 245, 203, 30, 255, 245, 203, 30, 255, 245, 203, 30, 255, 245, 203, 30, 255, 245, 203, 30, 255, 245, 203, 30, 255, 245, 203, 30, 255, 245, 203, 30, 255, 245, 203, 30, 254, 243, 201, 28, 254, 243, 201, 28, 255, 244, 201, 28, 255, 244, 201, 28, 255, 244, 201, 28, 255, 244, 201, 28, 255, 244, 201, 28, 255, 244, 201, 28, 255, 244, 201, 28, 255, 244, 201, 28, 255, 244, 201, 28, 255, 244, 201, 28, 255, 244, 201, 28, 255, 244, 201, 28, 254, 243, 201, 28, 254, 243, 201, 28, 253, 241, 198, 26, 254, 242, 199, 26, 255, 242, 199, 26, 255, 242, 199, 26, 255, 242, 199, 26, 255, 242, 199, 26, 255, 242, 199, 26, 255, 242, 199, 26, 255, 242, 199, 26, 255, 242, 199, 26, 255, 242, 199, 26, 255, 242, 199, 26, 255, 242, 199, 26, 255, 242, 199, 26, 254, 242, 199, 26, 253, 241, 198, 26, 174, 207, 171, 25, 252, 228, 188, 25, 252, 229, 188, 25, 252, 229, 188, 25, 252, 229, 188, 25, 252, 229, 188, 25, 252, 229, 188, 25, 252, 229, 188, 25, 252, 229, 188, 25, 252, 229, 188, 25, 252, 229, 188, 25, 252, 229, 188, 25, 252, 229, 188, 25, 252, 229, 188, 25, 252, 228, 188, 25, 174, 209, 172, 25, 1, 31, 25, 4, 19, 64, 53, 8, 21, 64, 53, 8, 21, 64, 53, 8, 21, 64, 53, 8, 21, 64, 53, 8, 21, 64, 53, 8, 21, 64, 53, 8, 21, 64, 53, 8, 21, 64, 53, 8, 21, 64, 53, 8, 21, 64, 53, 8, 21, 64, 53, 8, 21, 64, 53, 8, 19, 64, 53, 8, 1, 33, 27, 4, 0, 0, 0, 0, 0, 0, 0, 0, 0, 1, 0, 0, 0, 1, 0, 0, 0, 1, 0, 0, 0, 1, 0, 0, 0, 1, 0, 0, 0, 1, 0, 0, 0, 1, 0, 0, 0, 1, 0, 0, 0, 1, 0, 0, 0, 1, 0, 0, 0, 1, 0, 0, 0, 1, 0, 0, 0, 0, 0, 0, 0, 0, 0, 0], "mask"=[0, 0, 0, 0, 0, 127, 255, 255, 255, 255, 255, 255, 255, 255, 255, 255, 255, 255, 255, 255, 255, 255, 255, 255, 255, 255, 255, 255, 0, 0, 0, 0], "colors"=[], "Rectangle"={"left"=0, "top"=0, "right"=16, "bottom"=16}}  # Folder
        w140 = T6."Disabled and Grayed Out" ("Disabled")
        w141 = T6."Enabled" ("Disabled")
        # "Initialize the User Interface, here.\n(this is called automatically, by the Macro: Init)"
        n53 = invoke on="Menu Configuration" class="Tree (strict)" method="Edit Tree Items.Delete"(error in=w142) -> ()  [unwired: 4 in, 5 out]
        n54 = property on="Load" class="Bool"("DisabledEnum"=w141) -> ()  [unwired: 2 in, 2 out]
        n55 = property on="New" class="Bool"("DisabledEnum"=w141) -> ()  [unwired: 2 in, 2 out]
        n56 = property on="Edit" class="Bool"("DisabledEnum"=w140) -> ()  [unwired: 2 in, 2 out]
        n57 = property on="Save" class="Bool"("DisabledEnum"=w140) -> ()  [unwired: 2 in, 2 out]
        n58 = property on="Delete" class="Bool"("DisabledEnum"=w140) -> ()  [unwired: 2 in, 2 out]
        n59 = property on="Add" class="Bool"("DisabledEnum"=w140) -> ()  [unwired: 2 in, 2 out]
        n60 = Build Array(w139, w137, w136) -> (w138:T10[])
        n61 = for {
          tunnel: w138 -> [w149] mode=indexing
          i -> [w148]
          n62 = Add(x=40, y=w148) -> (x+y=w146:i32)
          n63 = invoke on="Menu Configuration" class="Tree (strict)" method="Custom Item Symbols.Set Symbol"("index"=w146, "image"=w149) -> ()  [unwired: 3 in, 5 out]
        }
        n64 = property on="Pane" class="Pane"("Origin"=T4 {"Horizontal"=0, "Vertical"=0}) -> ()  [unwired: 2 in, 2 out]
        n65 = call <vilib>:"Add State(s) to Queue__JKI_lib_State_Machine.vi"("State(s) in (\"\")"=w145) -> ("States Out"=w144:string)  [unwired: 14 in]
      }
      frame "UI: Cursor Set" {
        # "Argument"
        # "Set and Unset Cursor Busy.\n(Usage: \"UI: Cursor Set >> Busy|Idle\")"
        n66 = case shown="\"Idle\", Default" w150 {
          tunnel: w152 -> [w157 w159]
          tunnel: [w156 w158] -> w151
          frame "Idle", Default {
            n67 = call <vilib>:"Unset Busy.vi"("error in (no error)"=w157) -> ("error out"=w156:errorcluster)  [unwired: 10 in]
          }
          frame "Busy" {
            n68 = call <vilib>:"Set Busy.vi"("error in (no error)"=w159) -> ("error out"=w158:errorcluster)  [unwired: 9 in, 1 out]
          }
        }
        n69 = call <vilib>:"Add State(s) to Queue__JKI_lib_State_Machine.vi"("State(s) in (\"\")"=w155) -> ("States Out"=w154:string)  [unwired: 14 in]
      }
      frame "UI: Front Panel State" {
        # "Argument"
        # "Set Front Panel Open or Closed\n(Usage: \"UI: Front Panel State >> Open|Close\")"
        n70 = Unbundle By Name(w162) -> ("Core.Current VI Reference"=w161:refnum<vi>)
        n71 = case shown="\"Minimize\", \"Minimized\"" w160 {
          tunnel: w164 -> [w172 w187 w198 w211 w224]
          tunnel: [w174 w188 w200 w213 w226] -> w163
          tunnel: w161 -> [w173 w185 w199 w212 w225]
          frame "Open", "Standard", Default {
            w167 = T1."Standard" ("State")
            n72 = property class="VI"(reference=w173, error in=w172) -> (reference out=w170:refnum<vi>, error out=w171:errorcluster, "FP.State"=w169:T1)
            n73 = Not Equal?(x=w169, y=w167) -> (x != y?=w168:bool)
            n74 = case shown="True" w168 {
              tunnel: [w178 w180] -> w174
              tunnel: w171 -> [w177 w180]
              tunnel: w170 -> [w176 _]
              tunnel: w167 -> [w175 _]
              frame True {
                n75 = invoke class="VI" method="FP.Open"(reference=w176, error in=w177, "Activate"=TRUE, "State"=w175) -> (error out=w178:errorcluster)  [unwired: 1 in, 4 out]
              }
              frame False {
              }
            }
          }
          frame "Close", "Closed" {
            n76 = property class="VI"(reference=w185, error in=w187) -> (reference out=w184:refnum<vi>, error out=w186:errorcluster, "FP.State"=w182:T1)
            n77 = Not Equal?(x=w182, y=T1."Closed" ("Front Panel Window:State")) -> (x != y?=w181:bool)
            n78 = case shown="True" w181 {
              tunnel: [w189 w192] -> w188
              tunnel: w186 -> [w189 w191]
              tunnel: w184 -> [_ w190]
              frame False {
              }
              frame True {
                n79 = invoke class="VI" method="FP.Close"(reference=w190, error in=w191) -> (error out=w192:errorcluster)  [unwired: 1 in, 2 out]
              }
            }
          }
          frame "Hidden", "Hide" {
            w193 = T1."Hidden" ("State")
            n80 = property class="VI"(reference=w199, error in=w198) -> (reference out=w196:refnum<vi>, error out=w197:errorcluster, "FP.State"=w195:T1)
            n81 = Not Equal?(x=w195, y=w193) -> (x != y?=w194:bool)
            n82 = case shown="True" w194 {
              tunnel: [w204 w205] -> w200
              tunnel: w197 -> [w203 w205]
              tunnel: w196 -> [w202 _]
              tunnel: w193 -> [w201 _]
              frame True {
                n83 = invoke class="VI" method="FP.Open"(reference=w202, error in=w203, "State"=w201) -> (error out=w204:errorcluster)  [unwired: 2 in, 4 out]
              }
              frame False {
              }
            }
          }
          frame "Minimize", "Minimized" {
            w206 = T1."Minimized" ("State")
            n84 = property class="VI"(reference=w212, error in=w211) -> (reference out=w209:refnum<vi>, error out=w210:errorcluster, "FP.State"=w208:T1)
            n85 = Not Equal?(x=w208, y=w206) -> (x != y?=w207:bool)
            n86 = case shown="True" w207 {
              tunnel: [w217 w218] -> w213
              tunnel: w210 -> [w216 w218]
              tunnel: w209 -> [w215 _]
              tunnel: w206 -> [w214 _]
              frame True {
                n87 = invoke class="VI" method="FP.Open"(reference=w215, error in=w216, "State"=w214) -> (error out=w217:errorcluster)  [unwired: 2 in, 4 out]
              }
              frame False {
              }
            }
          }
          frame "Maximize", "Maximized" {
            w219 = T1."Maximized" ("State")
            n88 = property class="VI"(reference=w225, error in=w224) -> (reference out=w222:refnum<vi>, error out=w223:errorcluster, "FP.State"=w221:T1)
            n89 = Not Equal?(x=w221, y=w219) -> (x != y?=w220:bool)
            n90 = case shown="True" w220 {
              tunnel: [w230 w231] -> w226
              tunnel: w223 -> [w229 w231]
              tunnel: w222 -> [w228 _]
              tunnel: w219 -> [w227 _]
              frame True {
                n91 = invoke class="VI" method="FP.Open"(reference=w228, error in=w229, "State"=w227) -> (error out=w230:errorcluster)  [unwired: 2 in, 4 out]
              }
              frame False {
              }
            }
          }
        }
        n92 = call <vilib>:"Add State(s) to Queue__JKI_lib_State_Machine.vi"("State(s) in (\"\")"=w166) -> ("States Out"=w165:string)  [unwired: 14 in]
      }
      frame "---------- Macro ----------" {
        # "Do not put any code in this frame.\n(It is a separator no-op. You can make a copy of this frame to create a new Macro frame)"
        n93 = call <vilib>:"Add State(s) to Queue__JKI_lib_State_Machine.vi"("State(s) in (\"\")"=w235) -> ("States Out"=w234:string)  [unwired: 14 in]
      }
      frame "Macro: Initialize" {
        w236 = "Data: Initialize\nInitialize Core Data\nUI: Initialize\nUI: Front Panel State >> Open"  # Data: Initialize Initialize Core Data UI: Initialize UI: Front Panel State >> Open
        # "Initialization Macro\n(This is called once, when the VI starts)"
        n94 = call <vilib>:"Add State(s) to Queue__JKI_lib_State_Machine.vi"("State(s) in Front (\"\")"=w236, "State(s) in (\"\")"=w240) -> ("States Out"=w239:string)  [unwired: 13 in]
      }
      frame "Macro: Exit" {
        # "Exit Macro\n(This is called once, when the VI exits)"
        n95 = Unbundle By Name(w247) -> ("Core.Close Panel on Exit?"=w246:bool)
        n96 = Select(t="UI: Front Panel State >> Close", s=w246, f="") -> (s? t:f=w243:string)
        n97 = call <vilib>:"Add State(s) to Queue__JKI_lib_State_Machine.vi"("State(s) in (\"\")"=w243, "State(s) at Back (\"\")"="Data: Cleanup\nExit") -> ("States Out"=w241:string)  [unwired: 13 in]
        n98 = call <vilib>:"Add State(s) to Queue__JKI_lib_State_Machine.vi"("State(s) in Front (\"\")"=w241, "State(s) in (\"\")"=w250) -> ("States Out"=w249:string)  [unwired: 13 in]
      }
      frame "---------- Button Options ----------" {
        # "Template Separator\n(You can make a copy of, or modify, this frame)"
        n99 = call <vilib>:"Add State(s) to Queue__JKI_lib_State_Machine.vi"("State(s) in (\"\")"=w254) -> ("States Out"=w253:string)  [unwired: 14 in]
      }
      frame "Button Options: Load" {
        # "Your code here.\n(You can make a copy of, or modify, this frame)"
        n100 = Unbundle By Name(w257) -> ("SyncSols Menu"=w256:T3)
        n101 = call "File Dialog"("prompt"="Select SyncSols Menu File", "pattern (all files)"="*.smenu") -> ("selected path"=w255:path, "cancelled"=w259:bool, "error out"=w258:errorcluster)  [unwired: 10 in, 1 out]
        n102 = case shown="False" w259 {
          tunnel: w255 -> [w272 _]
          tunnel: w265 -> [w271 w274]
          tunnel: [w269 w274] -> w264
          tunnel: [w268 w273] -> w260
          tunnel: w258 -> [_ _]
          tunnel: w256 -> [_ w273]
          frame False {
            n103 = Read from Text File(file (use dialog)=w272, error in=w271) -> (text=w270:string, error out=w269:errorcluster)  [unwired: 2 in, 2 out]
            n104 = call <vilib>:"Tree Map from Pretty XML.vi"("Pretty XML"=w270) -> ("Tree Map Out"=w268:T3)  [unwired: 9 in, 1 out]
          }
          frame True {
          }
        }
        n105 = Bundle By Name(cluster=w257, "Current Path"=w255, "SyncSols Menu"=w260) -> (w261:T8)
        n106 = call <vilib>:"Add State(s) to Queue__JKI_lib_State_Machine.vi"("State(s) in (\"\")"=w267) -> ("States Out"=w266:string)  [unwired: 14 in]
      }
      frame "Button Options: New" {
        n107 = call "File Dialog2"("prompt"="Create New Menu File", "button label"="Create", "pattern (all files)"="*.smenu") -> ("selected path"=w275:path, "cancelled"=w280:bool, "error out"=w279:errorcluster)  [unwired: 9 in, 1 out]
        n108 = case shown="False" w280 {
          tunnel: w275 -> [w297 _]
          tunnel: w281 -> [w295 _]
          tunnel: w279 -> [_ _]
          tunnel: string[] ["Button_Color_Off", "Button_Color_On", "Button_Label_Color", "Extend_Sub_Menu_Icon", "Panel_Color"] ("New Root Name") -> [w289 _]
          tunnel: [w288 T3 {} ("Tree Map Out")] -> w276
          frame False {
            n109 = Open/Create/Replace File(file path (use dialog)=w297, error in=w295, operation (0:open)=T5."create") -> (refnum out=w293:refnum<file>, error out=w294:errorcluster)  [unwired: 3 in, 1 out]
            n110 = Close File(refnum=w293, error in=w294) -> ()  [unwired: 2 out]
            n111 = call <vilib>:"Add Root.vi"("New Root Name"="Menu_Configuration") -> ("Tree Map Out"=w292:T3, "Root Path"=w290:string)  [unwired: 9 in]
            n112 = for {
              tunnel: w290 -> [w301]
              shift-right: [w300] -> w288
              shift-left: w292 -> [w302]
              tunnel: w289 -> [w299] mode=indexing
              n113 = call <vilib>:"Add Node.vi"("Parent Path"=w301, "Data"="0", "New Node Name"=w299, "Tree Map In"=w302) -> ("Tree Map Out"=w300:T3)  [unwired: 5 in, 2 out]
            }
          }
          frame True {
          }
        }
        n114 = Bundle By Name(cluster=w285, "Current Path"=w275, "SyncSols Menu"=w276) -> (w277:T8)
        n115 = call <vilib>:"Add State(s) to Queue__JKI_lib_State_Machine.vi"("State(s) in (\"\")"=w287) -> ("States Out"=w286:string)  [unwired: 14 in]
      }
      frame "Button Options: Add" {
        n116 = Unbundle By Name(w323) -> ("Path"=w313:string, "SyncSols Menu"=w322:T3)
        n117 = Search and Replace String(replace all?=TRUE ("replace all? (F)"), input string=w313, search string="\\") -> (number of replacements=w309:i32)  [unwired: 5 in, 3 out]
        n118 = Decrement(x=w309) -> (x-1=w304:i32)
        n119 = call "Add New Menu Item Popup.vi"("error in"=w318) -> ("error out"=w305:errorcluster, "Path"=w316:string, "Label Out"=w314:string)  [unwired: 8 in]
        n120 = Index Array(array=string[] ["Root_Menu_Data", "Sub_Menu_Data", "Child_Menu_Data"], index=w304) -> (element=w308:string)
        n121 = call <vilib>:"Add Node.vi"("Parent Path"=w313, "New Node Name"=w308, "Tree Map In"=w322) -> ("Tree Map Out"=w321:T3, "New Node Path"=w320:string)  [unwired: 6 in, 1 out]
        n122 = call <vilib>:"Add Node.vi"("Parent Path"=w320, "Data"=w316, "New Node Name"="Button_Icon", "Tree Map In"=w321) -> ("Tree Map Out"=w319:T3)  [unwired: 5 in, 2 out]
        n123 = call <vilib>:"Add Node.vi"("Parent Path"=w320, "Data"=w314, "New Node Name"="Button_Label", "Tree Map In"=w319) -> ("Tree Map Out"=w306:T3)  [unwired: 5 in, 2 out]
        n124 = Bundle By Name(cluster=w323, "SyncSols Menu"=w306) -> (w307:T8)
        n125 = call <vilib>:"Add State(s) to Queue__JKI_lib_State_Machine.vi"("State(s) in (\"\")"=w325) -> ("States Out"=w324:string)  [unwired: 14 in]
      }
      frame "Button Options: Edit" {
        n126 = Unbundle By Name(w336) -> ("Selected Tag"=w335:string, "Data"=w327:string)
        n127 = call "Launch Edit Popup.vi"("error in"=w334, "Data"=w327, "Selected Tag"=w335) -> ("error out"=w333:errorcluster, "Data Out"=w326:string)  [unwired: 7 in]
        n128 = Not Equal?(x=w327, y=w326) -> (x != y?=w332:bool)
        n129 = Bundle By Name(cluster=w336, "Data"=w326) -> (w328:T8)
        n130 = Select(t="Tree Map: Update Data\nTree Operation: Update", s=w332, f="") -> (s? t:f=w329:string)
        n131 = call <vilib>:"Add State(s) to Queue__JKI_lib_State_Machine.vi"("State(s) in (\"\")"=w338, "State(s) at Back (\"\")"=w329) -> ("States Out"=w337:string)  [unwired: 13 in]
      }
      frame "Button Options: Delete" {
        n132 = Unbundle By Name(w343) -> ("Path"=w341:string, "SyncSols Menu"=w342:T3)
        n133 = call <vilib>:"Remove Node.vi"("Node Path"=w341, "Tree Map In"=w342) -> ("Tree Map Out"=w339:T3)  [unwired: 7 in, 2 out]
        n134 = Bundle By Name(cluster=w343, "SyncSols Menu"=w339) -> (w340:T8)
        n135 = call <vilib>:"Add State(s) to Queue__JKI_lib_State_Machine.vi"("State(s) in (\"\")"=w346) -> ("States Out"=w345:string)  [unwired: 14 in]
      }
      frame "Button Options: Save" {
        # "Template Separator\n(You can make a copy of, or modify, this frame)"
        n136 = Unbundle By Name(w352) -> ("Current Path"=w349:path, "SyncSols Menu"=w351:T3)
        n137 = call <vilib>:"Tree Map to Pretty XML.vi"("Root Path"="\\Menu_Configuration", "Tree Map In"=w351) -> ("Pretty XML"=w350:string)  [unwired: 8 in, 1 out]
        n138 = Write to Text File(file (use dialog)=w349, text=w350, error in=w348) -> ()  [unwired: 1 in, 3 out]
        n139 = call <vilib>:"Add State(s) to Queue__JKI_lib_State_Machine.vi"("State(s) in (\"\")"=w354) -> ("States Out"=w353:string)  [unwired: 14 in]
      }
      frame "Button Options: Enable/Options" {
        w360 = T6."Enabled" ("Disabled")
        w361 = T6."Disabled and Grayed Out" ("f")
        # "Template Separator\n(You can make a copy of, or modify, this frame)"
        n140 = Unbundle By Name(w372) -> ("Data Node?"=w363:bool, "Path"=w368:string)
        n141 = Search and Replace String(replace all?=TRUE ("replace all? (F)"), input string=w368, search string="\\") -> (number of replacements=w358:i32)  [unwired: 5 in, 3 out]
        n142 = Equal?(x=4, y=w358) -> (x = y?=w355:bool)
        n143 = Equal?(x=w358, y=1) -> (x = y?=w364:bool)
        n144 = Or(x=w363, y=w364) -> (x .or. y?=w362:bool)
        n145 = Or(x=w363, y=w355) -> (x .or. y?=w356:bool)
        n146 = Select(t=T6."Enabled" ("Disabled"), s=w363, f=w361) -> (s? t:f=w370:T6)
        n147 = Select(t=w361, s=w356, f=w360) -> (s? t:f=w369:T6)
        n148 = Select(t=w361, s=w362, f=w360) -> (s? t:f=w359:T6)
        n149 = property on="Edit" class="Bool"("DisabledEnum"=w370) -> ()  [unwired: 2 in, 2 out]
        n150 = property on="Add" class="Bool"("DisabledEnum"=w369) -> ()  [unwired: 2 in, 2 out]
        n151 = property on="Delete" class="Bool"("DisabledEnum"=w359) -> ()  [unwired: 2 in, 2 out]
        n152 = call <vilib>:"Add State(s) to Queue__JKI_lib_State_Machine.vi"("State(s) in (\"\")"=w375) -> ("States Out"=w374:string)  [unwired: 14 in]
      }
      frame "---------- Tree Operation ----------" {
        # "Template Separator\n(You can make a copy of, or modify, this frame)"
        n153 = call <vilib>:"Add State(s) to Queue__JKI_lib_State_Machine.vi"("State(s) in (\"\")"=w379) -> ("States Out"=w378:string)  [unwired: 14 in]
      }
      frame "Tree Operation: Update" {
        # "Template Separator\n(You can make a copy of, or modify, this frame)"
        n154 = Unbundle By Name(w389) -> ("SyncSols Menu"=w388:T3)
        n155 = call <vilib>:"Tree Map to Tree Control Items.vi"("Tree Map In"=w388) -> ("Tree Control Items"=w386:T11)  [unwired: 10 in]
        n156 = call "Update Tree Item Symbol and Clolor.vi"("error in"=w385, "Tree Control Items"=w386) -> ("error out"=w384:errorcluster, "Tree Control ItemsOut"=w382:T11)  [unwired: 8 in]
        n157 = invoke on="Menu Configuration" class="Tree (strict)" method="Edit Tree Items.Delete"(error in=w384) -> (error out=w387:errorcluster)  [unwired: 4 in, 4 out]
        n158 = control-ref of="Menu Configuration"() -> (w381:refnum<vi>)
        n159 = invoke on="Menu Configuration" class="Tree (strict)" method="Edit Tree Items.Add Multiple Items to End"(error in=w387, "Items"=w382) -> (error out=w383:errorcluster)  [unwired: 2 in, 3 out]
        n160 = call "Update Tree Item Symbol and Clolor.vi"("Tree Refnum"=w381, "error in"=w383, "Tree Control Items"=w382) -> ("error out"=w380:errorcluster)  [unwired: 7 in, 1 out]
        n161 = call <vilib>:"Add State(s) to Queue__JKI_lib_State_Machine.vi"("State(s) in (\"\")"=w391) -> ("States Out"=w390:string)  [unwired: 14 in]
      }
      frame "Tree Operation: Value Change" {
        # "Template Separator\n(You can make a copy of, or modify, this frame)"
        n162 = Unbundle By Name(w401) -> ("SyncSols Menu"=w398:T3)
        n163 = invoke on="Menu Configuration" class="Tree (strict)" method="Navigate Tree.Get Path"("tag"="Menu Configuration") -> ("Navigate Tree:Get Path"=w400:string[])  [unwired: 3 in, 3 out]
        n164 = Delete From Array(array=w400) -> (deleted portion=w394:string)  [unwired: 2 in, 1 out]
        n165 = Look In Map(map=w398, key=w394) -> (value=w399:T12)  [unwired: 1 in, 1 out]
        n166 = Unbundle By Name(w399) -> ("Data"=w393:string)
        n167 = Empty String/Path?(string/path=w393) -> (empty?=w397:bool)
        n168 = Not(x=w397) -> (.not. x?=w395:bool)
        n169 = Bundle By Name(cluster=w401, "Data Node?"=w395, "Path"=w394, "Data"=w393, "Selected Tag"="Menu Configuration") -> (w396:T8)
        n170 = call <vilib>:"Add State(s) to Queue__JKI_lib_State_Machine.vi"("State(s) in (\"\")"=w404) -> ("States Out"=w403:string)  [unwired: 14 in]
      }
      frame "---------- Tree Map ----------" {
        # "Template Separator\n(You can make a copy of, or modify, this frame)"
        n171 = call <vilib>:"Add State(s) to Queue__JKI_lib_State_Machine.vi"("State(s) in (\"\")"=w408) -> ("States Out"=w407:string)  [unwired: 14 in]
      }
      frame "Tree Map: Update Data" {
        # "Template Separator\n(You can make a copy of, or modify, this frame)"
        n172 = Unbundle By Name(w415) -> ("SyncSols Menu"=w414:T3, "Path"=w413:string, "Data"=w412:string)
        n173 = in-place {
          in-place-border: w412 -> [w419]
          n174 = in-place-map #1(w414, w413) -> (w422:T12)  [unwired: 1 in, 1 out]
          n175 = Bundle By Name(cluster=w422, "Data"=w419) -> (w421:T12)
          n176 = in-place-map #1(w421, LVMapReplaceAction."Modify Entry only if found" ("action")) -> (w410:T3)  [unwired: 2 out]
        }
        n177 = property on="Save" class="Bool"("DisabledEnum"=T6."Enabled" ("Disabled")) -> ()  [unwired: 2 in, 2 out]
        n178 = Bundle By Name(cluster=w415, "SyncSols Menu"=w410) -> (w411:T8)
        n179 = call <vilib>:"Add State(s) to Queue__JKI_lib_State_Machine.vi"("State(s) in (\"\")"=w418) -> ("States Out"=w417:string)  [unwired: 14 in]
      }
    }
  }
